vi "Destroy All Channels.vi"(8 "error in (no error)":errorcluster, 11 "CIFChannelMng in":refnum<class "CIFChannelMng.lvclass">) -> (0 "error out":errorcluster, 3 "CIFChannelMng out":refnum<class "CIFChannelMng.lvclass">)   [LabVIEW 2021, in "CIFChannelMng.lvclass"]
uses:
  CIFChannelMng.lvclass
  CIFChannelMng.lvclass/CIFChannelMng.ctl
  <vilib>/CIF Foundation/CIF Channels Core/CIFChannels/CIFChannels.lvclass/CIFChannels.ctl
  Accessors/Read Channel Array.vi
  <vilib>/CIF Foundation/CIF Channels Core/ChannelCommon/Utilities/Add Error.vi
  <vilib>/CIF Foundation/CIF Channels Core/CIFChannels/Accessors/Read Name.vi
  <vilib>/CIF Foundation/CIF Channels Core/CIFChannels/Accessors/Write Channel State.vi
  <vilib>/CIF Foundation/CIF Utilities/Errors/Append Error Location.vi
  <vilib>/CIF Foundation/CIF Channels Core/CIFChannels/CIFChannels.lvclass
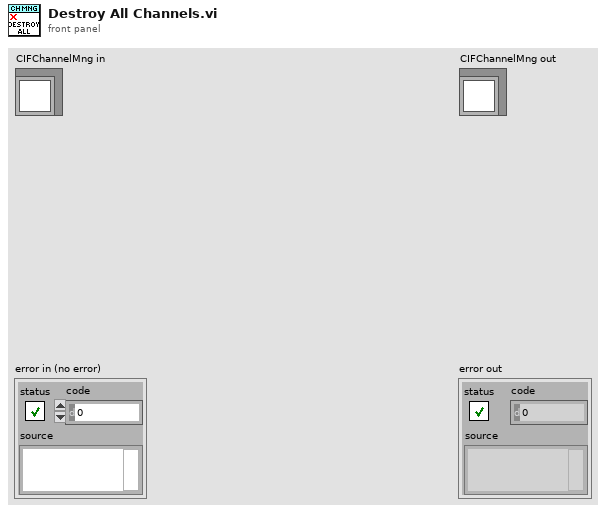
[diagram p1: front panel]
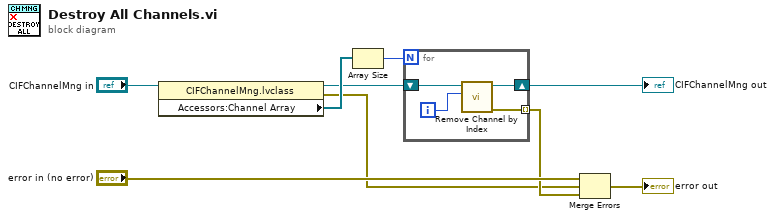
[diagram p0: block diagram]
diagram:
  n1 = property class="CIFChannelMng.lvclass"(reference="CIFChannelMng in") -> (reference out=w4:refnum<class "CIFChannelMng.lvclass">, error out=w1:errorcluster, "Accessors:Channel Array"=w7:refnum<class "CIFChannels.lvclass">[])  [unwired: 1 in]
  n2 = Array Size(array=w7) -> (size(s)=w5:i32)
  n3 = for {
    N: w5 -> [_]
    shift-right: [w11] -> w3
    shift-left: w4 -> [w13]
    tunnel: [w10] -> w2 mode=indexing
    i -> [w12]
    n4 = call "Remove Channel by Index.vi"("Channel Index"=w12, "CIFChannelMng in"=w13) -> ("error out"=w10:errorcluster, "CIFChannelMng out"=w11:refnum<class "CIFChannelMng.lvclass">)  [unwired: 8 in]
  }
  "CIFChannelMng out" <- w3
  n5 = Merge Errors("error in (no error)", w1, w2) -> (→"error out":errorcluster)
